vi "SubViHelper.vi"(8 "error in (no error)":errorcluster caption="Fehler (Eingang, kein Fehler)") -> (0 "error out":errorcluster caption="Fehler (Ausgang)")   [LabVIEW 2013]
uses:
  PassDataAround/PassDataAround.lvclass
  LvDictionary/DictionaryClass/Dictionary.lvclass/Dictionary.ctl
  LvDictionary/DictionaryClass/Properties/GetDict.vi
  LvDictionary/DictionaryStringClass/DictionaryString.lvclass
panel:
  out "Dict 2":variant
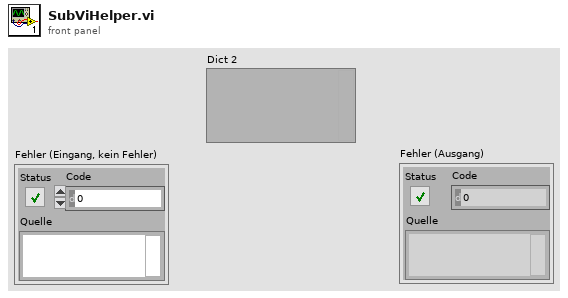
[diagram p1: front panel]
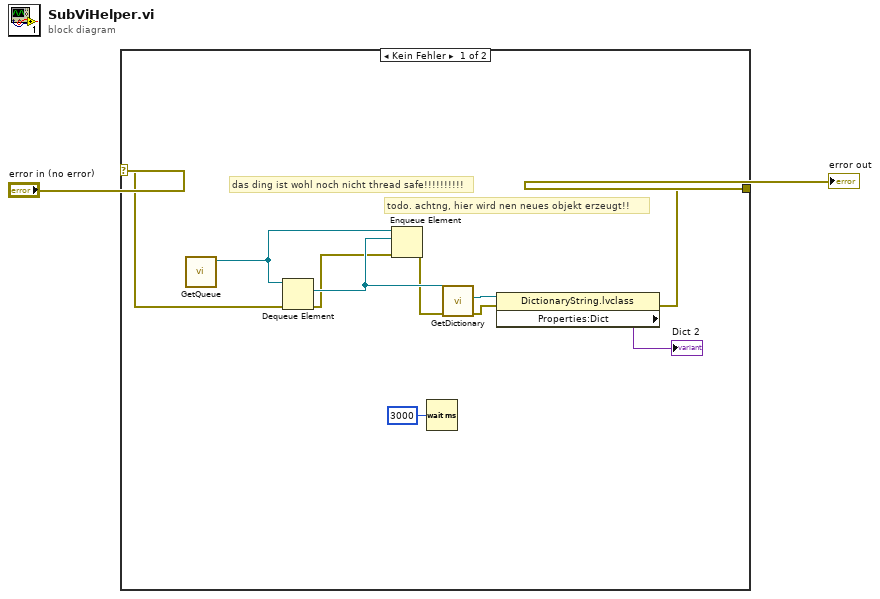
[diagram p0: block diagram]
diagram:
  n1 = case shown="Kein Fehler" "error in (no error)" {
    selector: "error in (no error)" -> [w9 w13]
    tunnel: [w8 w13] -> w1
    frame No Error {
      # "todo. achtng, hier wird nen neues objekt erzeugt!!"
      # "das ding ist wohl noch nicht thread safe!!!!!!!!!!"
      n2 = call "GetQueue.vi"() -> ("Singleton Queue"=w6:refnum<queue>)  [unwired: 10 in, 1 out]
      n3 = Dequeue Element(queue=w6, error in (no error)=w9) -> (element=w5:refnum<class "PassDataAround.lvclass">, error out=w4:errorcluster)  [unwired: 1 in, 2 out]
      n4 = Enqueue Element(queue=w6, element=w5, error in (no error)=w4) -> (error out=w3:errorcluster)  [unwired: 1 in, 2 out]
      n5 = Wait (ms)(milliseconds to wait=u32 3000 ("Zu wartende ms")) -> ()  [unwired: 1 out]
      n6 = call-dynamic "GetDictionary.vi"("error in (no error)"=w3, "PassDataAround Eingang"=w5) -> ("error out"=w11:errorcluster, "LvDictionary.lvlib:DictionaryString.lvclass"=w12:refnum<class "DictionaryString.lvclass">)  [unwired: 7 in, 1 out]
      n7 = property class="DictionaryString.lvclass"(reference=w12, error in=w11) -> (error out=w8:errorcluster, "Properties:Dict"=→"Dict 2":variant)  [unwired: 1 out]
    }
    frame Error {
    }
  }
  "error out" <- w1
